vi "ble_write_message_plus_wait.vi"(5 "Command Class (System)":T1 format="%02x" items=["System", "Persistent Store", "Attribute database", "Connection", "Attribute client", "Security Manager", "Generic Access Profile", "Hardware"], 7 "Message Type (Command / Response)":T2 format="%02x" items=["Command / Response"=0, "Event"=128], 8 "error in (no error)":errorcluster, 9 "Payload(Empty)":u8[](array[numeric]) format="%02x", 10 "Message ID (0x00)":u8 format="%02x", 11 "COM Bluegiga in":refnum<visa-resource-name>) -> (0 "error out":errorcluster, 2 "Data to Send":u8[](array[numeric]) format="%02x", 3 "COM Bluegiga out":refnum<visa-resource-name>)   [LabVIEW 2015]
uses:
  type_def/message_type.ctl
  type_def/message_class.ctl
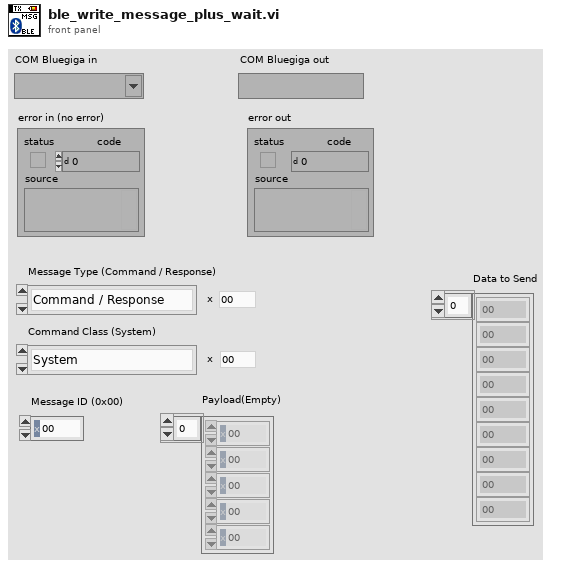
[diagram p1: front panel]
types:
  T1 = typedef "message_class.ctl" = u8
  T2 = typedef "message_type.ctl" = u8
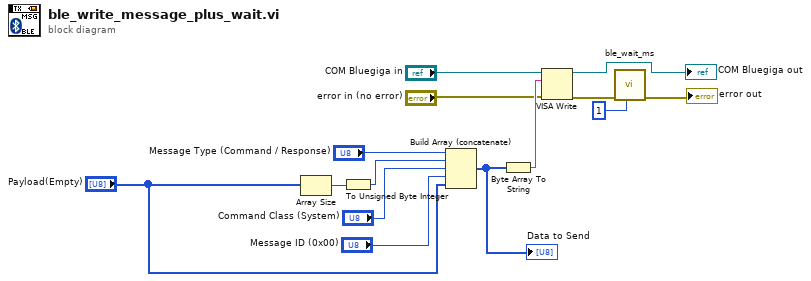
[diagram p0: block diagram]
diagram:
  n1 = Array Size(array="Payload(Empty)") -> (size(s)=w14:i32)
  n2 = To Unsigned Byte Integer(number=w14) -> (unsigned 8bit integer=w8:u8)
  n3 = Build Array (concatenate)("Message Type (Command / Response)", w8, "Command Class (System)", "Message ID (0x00)", "Payload(Empty)") -> (w9:T1[])
  "Data to Send" <- w9
  n4 = Byte Array To String(unsigned byte array=w9) -> (string=w13:string)
  n5 = VISA Write(VISA resource name="COM Bluegiga in", write buffer=w13, error in (no error)="error in (no error)") -> (VISA resource name out=→"COM Bluegiga out":refnum<visa-resource-name>, error out=w4:errorcluster)  [unwired: 1 out]
  n6 = call "ble_wait_ms.vi"("milliseconds to wait (100)"=u32 1, "error in (no error)"=w4) -> ("error out"=→"error out":errorcluster)  [unwired: 9 in]
